vi "Write Topic.vi"(8 "error in (no error)":errorcluster, 10 "Topic":string, 11 "CallResult JSON in":refnum<class "CallResult JSON.lvclass">) -> (0 "error out":errorcluster, 3 "CallResult JSON out":refnum<class "CallResult JSON.lvclass">)   [LabVIEW 2020, in "wamplv.lvlib" / "CallResult JSON.lvclass"]
uses:
  CallResult JSON.lvclass
  CallResult JSON.lvclass/CallResult JSON.ctl
  Message loop classes/ErrorOrSuccess JSON/ErrorOrSuccess JSON.lvclass
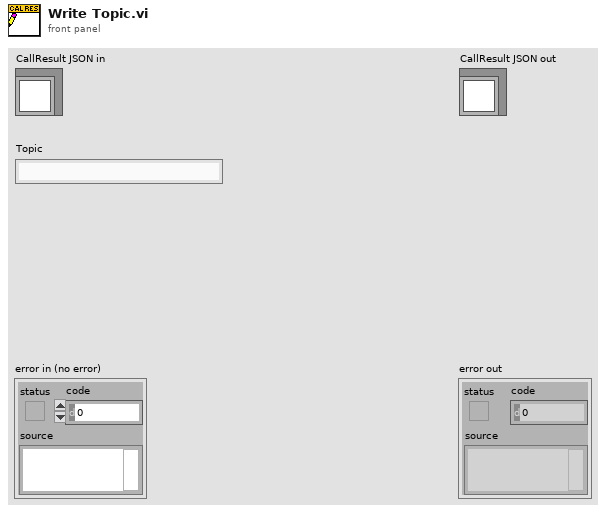
[diagram p1: front panel]
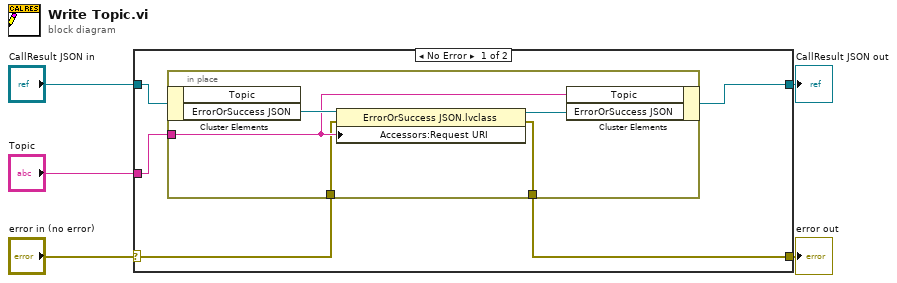
[diagram p0: block diagram]
diagram:
  n1 = case shown="No Error" "error in (no error)" {
    selector: "error in (no error)" -> [w7 w16]
    tunnel: [w6 w16] -> w4
    tunnel: [w9 w17] -> w2
    tunnel: "CallResult JSON in" -> [w10 w17]
    tunnel: "Topic" -> [w8 _]
    frame No Error {
      n2 = in-place {
        in-place-border: w8 -> [w13]
        in-place-border: w7 -> [w12]
        in-place-border: [w11] -> w6
        n3 = in-place-cluster #1(w10) -> ("ErrorOrSuccess JSON"=w15:refnum<class "ErrorOrSuccess JSON.lvclass">)  [unwired: 1 out]
        n4 = property class="ErrorOrSuccess JSON.lvclass"(reference=w15, error in=w12, "Accessors:Request URI"=w13) -> (reference out=w14:refnum<class "ErrorOrSuccess JSON.lvclass">, error out=w11:errorcluster)
        n5 = in-place-cluster #1("Topic"=w13, "ErrorOrSuccess JSON"=w14) -> (w9:refnum<class "CallResult JSON.lvclass">)
      }
    }
    frame Error {
    }
  }
  "error out" <- w4
  "CallResult JSON out" <- w2
